vi "Subscriber.vi"() -> ()   [LabVIEW 2022 SP3]
uses:
  <vilib>/LabVIEW Open Source Project/MQTT Client/Client class/Client.lvclass/Client.ctl
  <vilib>/LabVIEW Open Source Project/MQTT Connection/MQTT_Base/Base Class/MQTT_Base.lvclass/MQTT_Base.ctl
  <vilib>/LabVIEW Open Source Project/Connection/Connection.TCP/Connection.TCP.lvclass
  C:/Program Files/National Instruments/LabVIEW 2022/vi.lib/LabVIEW Open Source Project/Connection/Connection/Connection.lvclass
  <vilib>/LabVIEW Open Source Project/MQTT Client/Client class/Client.lvclass
  C:/Program Files/National Instruments/LabVIEW 2022/vi.lib/LabVIEW Open Source Project/MQTT Connection/MQTT_Base/Base Class/MQTT_Base.lvclass
  <vilib>/LabVIEW Open Source Project/MQTT Control Packets/Control Packets/PUBLISH/PUBLISH.lvclass
  <vilib>/LabVIEW Open Source Project/MQTT Connection/MQTT_Base/Base Class/MQTT_Base.lvclass
  <vilib>/LabVIEW Open Source Project/Connection/Connection.LocalQueue/Connection.LocalQueue.lvclass
  <vilib>/LabVIEW Open Source Project/Connection/Connection/Connection.lvclass
  C:/Program Files/National Instruments/LabVIEW 2022/vi.lib/LabVIEW Open Source Project/MQTT Client/Client class/Client.lvclass
panel:
  out "Unsuback":bool
  out "Suback":bool
  in  "Subscribe":bool
  in  "Connection":bool
  in  "Stop Client":bool
  out "Waveform Chart":dbl(graph)
  out "last error":errorcluster
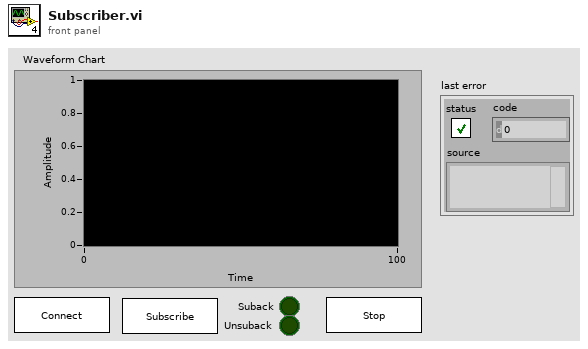
[diagram p1: front panel]
types:
  T1 = typedef "MQTT Client.lvlib/Client.lvclass/Public Events -- cluster.ctl" = cluster{"Connection Status":refnum<user-event>, "Connected":refnum<user-event>, "Application Message":refnum<user-event>}
  T2 = typedef "MQTT Base.lvlib/MQTT_Base.lvclass/Public Events -- cluster.ctl" = cluster{"Stop Event":refnum<user-event>, "Error Event":refnum<user-event>, "Inbound Message":refnum<user-event>}
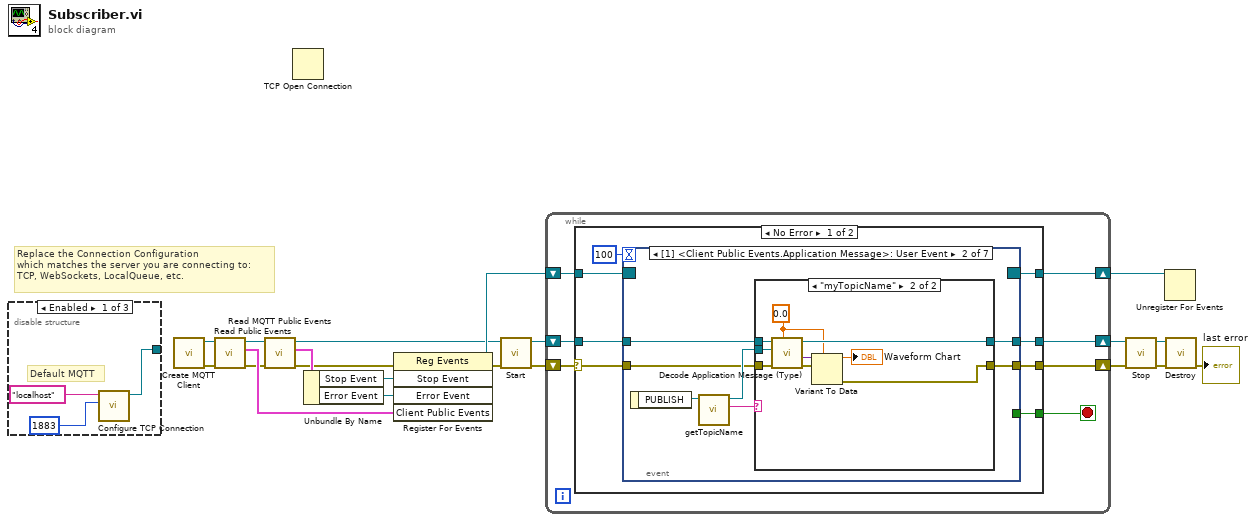
[diagram p0: block diagram]
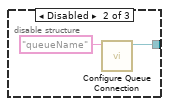
[diagram p2: hidden frame]
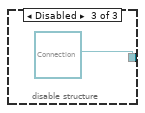
[diagram p3: hidden frame]
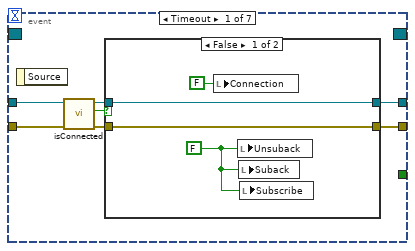
[diagram p4: hidden frame]
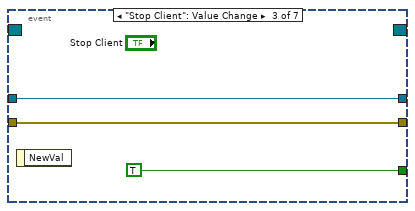
[diagram p7: hidden frame]
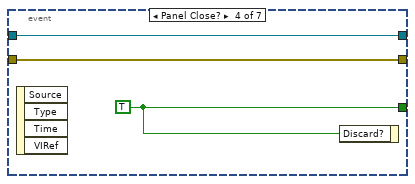
[diagram p8: hidden frame]
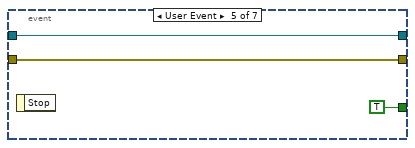
[diagram p9: hidden frame]
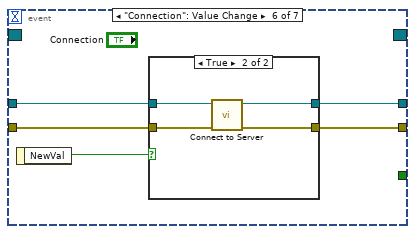
[diagram p10: hidden frame]
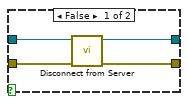
[diagram p11: hidden frame]
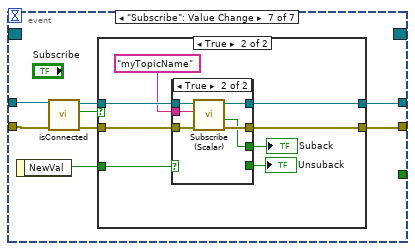
[diagram p12: hidden frame]
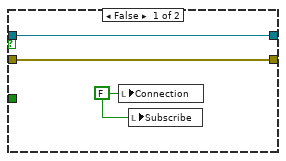
[diagram p13: hidden frame]
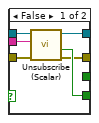
[diagram p14: hidden frame]
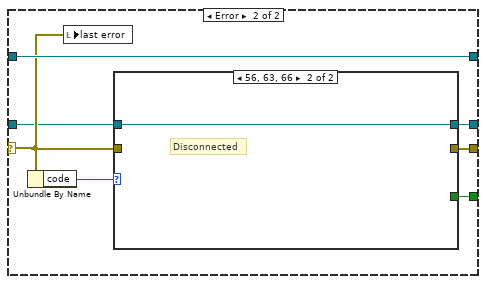
[diagram p15: hidden frame]
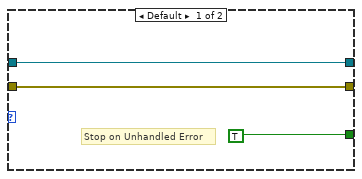
[diagram p16: hidden frame]
diagram:
  # "Replace the Connection Configuration\nwhich matches the server you are connecting to:\nTCP, WebSockets, LocalQueue, etc."
  n1 = disable-structure shown="Enabled" {
    disable-tunnel: [w22 w25 refnum<class "Connection.lvclass"> refnum ("Connection Configuration")] -> _
    frame Enabled {
      # "Default MQTT"
      n2 = call <vilib>:"Configure TCP Connection.vi"("remote port (80)"=u16 1883, "address (localhost)"="localhost") -> ("Connection.TCP"=w22:refnum<class "Connection.TCP.lvclass">)  [unwired: 8 in, 1 out]
    }
    frame Disabled {
      n3 = call <vilib>:"Configure Queue Connection.vi"("Queue Name"="queueName") -> ("Connection.LocalQueue"=w25:refnum<class "Connection.LocalQueue.lvclass">)  [unwired: 9 in, 1 out]
    }
    frame Disabled {
    }
  }
  n4 = call <vilib>:"Create MQTT Client.vi"() -> ("error out"=w3:errorcluster, "Client out"=w1:refnum<class "Client.lvclass">)  [unwired: 10 in]
  n5 = call <vilib>:"Read Public Events.vi"("error in (no error)"=w3, "Client in"=w1) -> ("error out"=w4:errorcluster, "Client Public Events"=w6:T1, "Client out"=w2:refnum<class "Client.lvclass">)  [unwired: 7 in]
  n6 = call <vilib>:"Read MQTT Public Events.vi"("error in (no error)"=w4, "MQTT_Base in"=w2) -> ("error out"=w5:errorcluster, "MQTT Public Events"=w13:T2, "MQTT_Base out"=w8:refnum<class "Client.lvclass">)  [unwired: 7 in]
  n7 = TCP Open Connection() -> ()  [unwired: 5 in, 2 out]
  n8 = Unbundle By Name(w13) -> ("Stop Event"=w11:refnum<user-event>, "Error Event"=w12:refnum<user-event>)
  n9 = register-events(error in=w5, w11, w12, w6) -> (reference out=w9:refnum<event-registration>, error out=w7:errorcluster)  [unwired: 1 in]
  n10 = call <vilib>:"Start.vi"("error in (no error)"=w7, "MQTT_Base in"=w8) -> ("error out"=w19:errorcluster, "MQTT_Base out"=w18:refnum<class "Client.lvclass">)  [unwired: 7 in, 1 out]
  n11 = while {
    shift-right: [w32] -> w10
    shift-left: w9 -> [w33]
    shift-right: [w29] -> w15
    shift-left: w18 -> [w30]
    shift-right: [w31] -> w17
    shift-left: w19 -> [w27]
    stop <- w28 stop-if-true
    n12 = case shown="No Error" w27 {
      selector: w27 -> [w34 w129]
      tunnel: w33 -> [w41 w132]
      tunnel: [w40 w132] -> w32
      tunnel: [w39 w127] -> w31
      tunnel: w30 -> [w37 w128]
      tunnel: [w36 w131] -> w29
      tunnel: [w35 w126] -> w28
      frame No Error {
        n13 = event shown="[1] <Client Public Events.Application Message>: User Event" {
          selector: w41 -> [_ _ _ _ _ _ _]
          dyn-events: [_ _ _ _ _ _ _] -> w40
          timeout: 100 -> [_ _ _ _ _ _ _]
          tunnel: w34 -> [w44 w58 w74 w76 w81 w82 w100]
          tunnel: [w47 w55 w74 w76 w81 w83 w101] -> w39
          tunnel: [_ _ TRUE w78 TRUE _ _] -> w35
          tunnel: w37 -> [w46 w59 w75 w77 w79 w86 w99]
          tunnel: [w48 w57 w75 w77 w79 w84 w102] -> w36
          event Timeout {
            n14 = event-data() -> ()  [unwired: 1 in, 1 out]
            n15 = call <vilib>:"isConnected.vi"("error in (no error)"=w44, "Client in"=w46) -> ("error out"=w43:errorcluster, "connected"=w42:bool, "Client out"=w45:refnum<class "Client.lvclass">)  [unwired: 7 in]
            n16 = case shown="False" w42 {
              tunnel: [w52 w54] -> w48
              tunnel: [w51 w53] -> w47
              tunnel: w45 -> [w52 w54]
              tunnel: w43 -> [w51 w53]
              frame False {
                w50 = FALSE
                n17 = local write "Connection"(FALSE ("Connection")) -> ()
                n18 = local write "Unsuback"(w50) -> ()
                n19 = local write "Suback"(w50) -> ()
                n20 = local write "Subscribe"(w50) -> ()
              }
              frame True {
              }
            }
          }
          event User Event {
            n21 = event-data() -> ("PUBLISH"=w61:refnum<class "PUBLISH.lvclass">)  [unwired: 1 in]
            n22 = call <vilib>:"getTopicName.vi"("PUBLISH in"=w61) -> ("Topic"=w56:string, "PUBLISH out"=w60:refnum<class "PUBLISH.lvclass">)  [unwired: 8 in, 1 out]
            n23 = case shown="\"myTopicName\"" w56 {
              tunnel: w60 -> [_ w64]
              tunnel: w59 -> [w63 w70]
              tunnel: w58 -> [w62 w68]
              tunnel: [w63 w69] -> w57
              tunnel: [w62 w72] -> w55
              frame Default {
              }
              frame "myTopicName" {
                w66 = 0.0
                n24 = call <vilib>:"Decode Application Message (Type).vi"("Type"=w66, "error in (no error)"=w68, "PUBLISH"=w64, "Client in"=w70) -> ("error out"=w67:errorcluster, "Payload"=w65:variant, "Client out"=w69:refnum<class "Client.lvclass">)  [unwired: 4 in, 1 out]
                n25 = Variant To Data(error in=w67, type=w66, Variant=w65) -> (data=→"Waveform Chart":dbl, error out=w72:errorcluster)
              }
            }
          }
          event "Stop Client": Value Change {
            n26 = event-data() -> ()  [unwired: 1 in, 1 out]
          }
          event Panel Close? {
            w78 = TRUE
            n27 = event-data() -> ()  [unwired: 1 in, 4 out]
            n28 = event-data("Discard?"=w78) -> ()  [unwired: 1 in, 1 out]
          }
          event User Event {
            n29 = event-data() -> ()  [unwired: 1 in, 1 out]
          }
          event "Connection": Value Change {
            n30 = event-data() -> ("NewVal"=w85:bool)  [unwired: 1 in]
            n31 = case shown="True" w85 {
              tunnel: w86 -> [w90 w94]
              tunnel: [w89 w91] -> w84
              tunnel: [w88 w92] -> w83
              tunnel: w82 -> [w87 w93]
              frame False {
                n32 = call <vilib>:"Disconnect from Server.vi"("error in (no error)"=w87, "Client in"=w90) -> ("error out"=w88:errorcluster, "Client out"=w89:refnum<class "Client.lvclass">)  [unwired: 7 in, 1 out]
              }
              frame True {
                n33 = call <vilib>:"Connect to Server.vi"("error in (no error)"=w93, "Client in"=w94) -> ("error out"=w92:errorcluster, "Client out"=w91:refnum<class "Client.lvclass">)  [unwired: 6 in, 2 out]
              }
            }
          }
          event "Subscribe": Value Change {
            n34 = event-data() -> ("NewVal"=w95:bool)  [unwired: 1 in]
            n35 = call <vilib>:"isConnected.vi"("error in (no error)"=w100, "Client in"=w99) -> ("error out"=w97:errorcluster, "connected"=w96:bool, "Client out"=w98:refnum<class "Client.lvclass">)  [unwired: 7 in]
            n36 = case shown="True" w96 {
              tunnel: [w105 w113] -> w102
              tunnel: [w104 w112] -> w101
              tunnel: w98 -> [w105 w111]
              tunnel: w97 -> [w104 w110]
              tunnel: w95 -> [_ w108]
              frame False {
                w103 = FALSE ("Connection")
                n37 = local write "Connection"(w103) -> ()
                n38 = local write "Subscribe"(w103) -> ()
              }
              frame True {
                n39 = case shown="True" w108 {
                  tunnel: [w114 w122] -> w113
                  tunnel: [w115 w121] -> w112
                  tunnel: w111 -> [w119 w125]
                  tunnel: w110 -> [w118 w124]
                  tunnel: "myTopicName" ("Topic Name (empty: Payload name)") -> [w117 w123]
                  tunnel: [_ w120] -> w107
                  tunnel: [w116 _] -> w106
                  frame False {
                    n40 = call <vilib>:"Unsubscribe (Scalar).vi"("error in (no error)"=w118, "Topic Filter"=w117, "Client in"=w119) -> ("error out"=w115:errorcluster, "Ack"=w116:bool, "Client out"=w114:refnum<class "Client.lvclass">)  [unwired: 6 in]
                  }
                  frame True {
                    n41 = call <vilib>:"Subscribe (Scalar).vi"("error in (no error)"=w124, "Topic Filter"=w123, "Client in"=w125) -> ("error out"=w121:errorcluster, "Ack"=w120:bool, "Client out"=w122:refnum<class "Client.lvclass">)  [unwired: 6 in]
                  }
                }
                "Unsuback" <- w106
                "Suback" <- w107
              }
            }
          }
        }
      }
      frame Error {
        n42 = Unbundle By Name(w129) -> ("code"=w130:i32)
        n43 = local write "last error"(w129) -> ()
        n44 = case shown="56, 63, 66" w130 {
          tunnel: w128 -> [w135 w136]
          tunnel: [w135 w136] -> w131
          tunnel: w129 -> [w134 _]
          tunnel: [w134 _] -> w127
          tunnel: [TRUE _] -> w126
          frame Default {
            # "Stop on Unhandled Error"
          }
          frame 56, 63, 66 {
            # "Disconnected"
          }
        }
      }
    }
  }
  n45 = call <vilib>:"Stop.vi"("error in (no error)"=w17, "MQTT_Base in"=w15) -> ("error out"=w16:errorcluster, "MQTT_Base out"=w14:refnum<class "Client.lvclass">)  [unwired: 7 in, 1 out]
  n46 = Unregister For Events(event registration refnum=w10) -> ()  [unwired: 1 in, 1 out]
  n47 = call <vilib>:"Destroy.vi"("error in (no error)"=w16, "MQTT_Base in"=w14) -> ("error out"=→"last error":errorcluster)  [unwired: 8 in, 1 out]
